vi "PickRobots.vi"(0 "object in":refnum<class "Play_v2.lvclass">, 2 "Game":refnum<class "Game.lvclass">, 5 "error in (no error)":errorcluster) -> (14 "object out":refnum<class "Play_v2.lvclass">, 16 "Robots":refnum<class "Robot.lvclass">[](array[class]), 19 "error out":errorcluster)   [LabVIEW 2023, in "Play_v2.lvclass"]
uses:
  Play_v2.lvclass
  Game_class/Game.lvclass
  Robot_class/Robot.lvclass
  Play_v2.lvclass/Play_v2.ctl
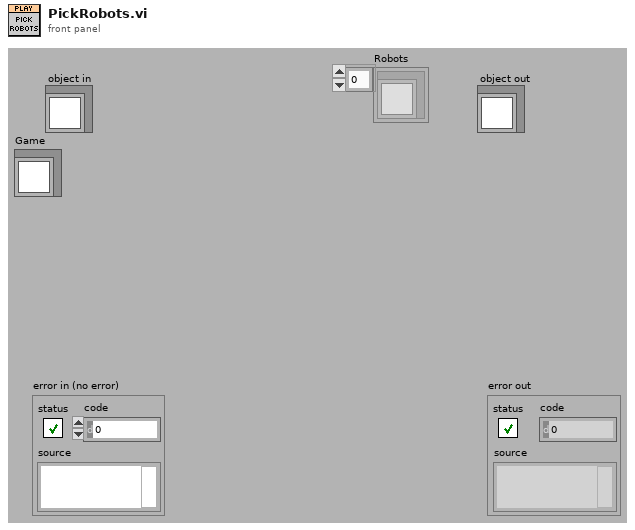
[diagram p1: front panel]
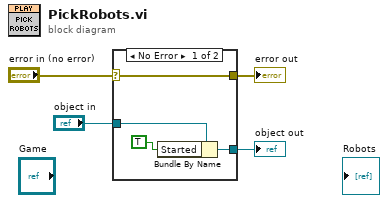
[diagram p0: block diagram]
diagram:
  n1 = case shown="No Error" "error in (no error)" {
    selector: "error in (no error)" -> [w8 w10]
    tunnel: [w8 w10] -> w3
    tunnel: [w5 w9] -> w1
    tunnel: "object in" -> [w7 w9]
    frame No Error {
      n2 = Bundle By Name(cluster=w7, "Started"=TRUE) -> (w5:refnum<class "Play_v2.lvclass">)
    }
    frame Error {
    }
  }
  "error out" <- w3
  "object out" <- w1
